vi "XLP80_Globals_Referenzen.vi"() -> ()   [LabVIEW 2021]
uses:
  XLP80_GUI_V001.llb/XLP80_GUI_TDefClusterPandID_Gen2_FM1.ctl
  XLP80_GUI_V001.llb/XLP80_GUI_TDefClusterPandID_Gen2_FM2.ctl
panel:
  in  "References":enum32{"Values", "ModeA", "Mode B", "Display"}(tab)
  in  "AI Values":refnum<vi>
  in  "DI Values":refnum<vi>
  in  "CAN WriteA Values":refnum<vi>
  in  "Listbox TestmodeA ReadCAN":refnum<vi>
  in  "Ref_CAN WriteA Names":refnum<vi>
  in  "Ref_Maxs Alarm":refnum<vi>
  in  "Ref_Names Alarm":refnum<vi>
  in  "Ref Listbox Alarm":refnum<vi>
  in  "Ref_Values Alarm":refnum<vi>
  in  "Ref_Units Alarm":refnum<vi>
  in  "Ref_Mins Alarm":refnum<vi>
  in  "Ref_Maxs Shutdown":refnum<vi>
  in  "Ref_Names Shutdown":refnum<vi>
  in  "Ref Listbox Shutdown":refnum<vi>
  in  "Ref_Values Shutdown":refnum<vi>
  in  "Ref_Units Shutdown":refnum<vi>
  in  "Ref_Mins Shutdown":refnum<vi>
  in  "Ref_Maxs Operational Mode":refnum<vi>
  in  "Ref_Names Operational Mode":refnum<vi>
  in  "Ref Listbox Operational Mode":refnum<vi>
  in  "Ref_Values Operational Mode":refnum<vi>
  in  "Ref_Units Operational Mode":refnum<vi>
  in  "Ref_Mins Operational Mode":refnum<vi>
  in  "Ref_Maxs Precond":refnum<vi>
  in  "Ref_Units Precond":refnum<vi>
  in  "Ref_Mins Precond":refnum<vi>
  in  "Ref_Names Precond":refnum<vi>
  in  "Ref_Values Precond":refnum<vi>
  in  "Ref_Maxs Power Management":refnum<vi>
  in  "Ref_Units Power Management":refnum<vi>
  in  "Ref_Mins Power Management":refnum<vi>
  in  "Ref_Maxs Basis Funktion":refnum<vi>
  in  "Ref_Units Basis Funktion":refnum<vi>
  in  "Ref_Mins Basis Funktion":refnum<vi>
  in  "Ref_Maxs HV&Software":refnum<vi>
  in  "Ref_Names Power Management":refnum<vi>
  in  "Ref Listbox Power Management":refnum<vi>
  in  "Ref_Values Power Management":refnum<vi>
  in  "Ref_Names Basis Funktion":refnum<vi>
  in  "Ref Listbox Basis Funktion":refnum<vi>
  in  "Ref_Values Basis Funktion":refnum<vi>
  in  "Ref_Names HV&Software":refnum<vi>
  in  "Ref Listbox HV&Software":refnum<vi>
  in  "Ref_Values HV&Software":refnum<vi>
  in  "Listbox TestmodeB ReadCAN":refnum<vi>
  in  "Ref_Units HV&Software":refnum<vi>
  in  "Ref_Mins HV&Software":refnum<vi>
  out "ExposureTime":refnum<vi>
  in  "P&ID_GEN2_FM1":refnum<vi>
  in  "Messages":refnum<vi>
  in  "GlobalStateTab":refnum<vi>
  in  "AutoTabCtl":refnum<vi>
  in  "ManTabCtl":refnum<vi>
  in  "P&ID_GEN2_FM2":refnum<vi>
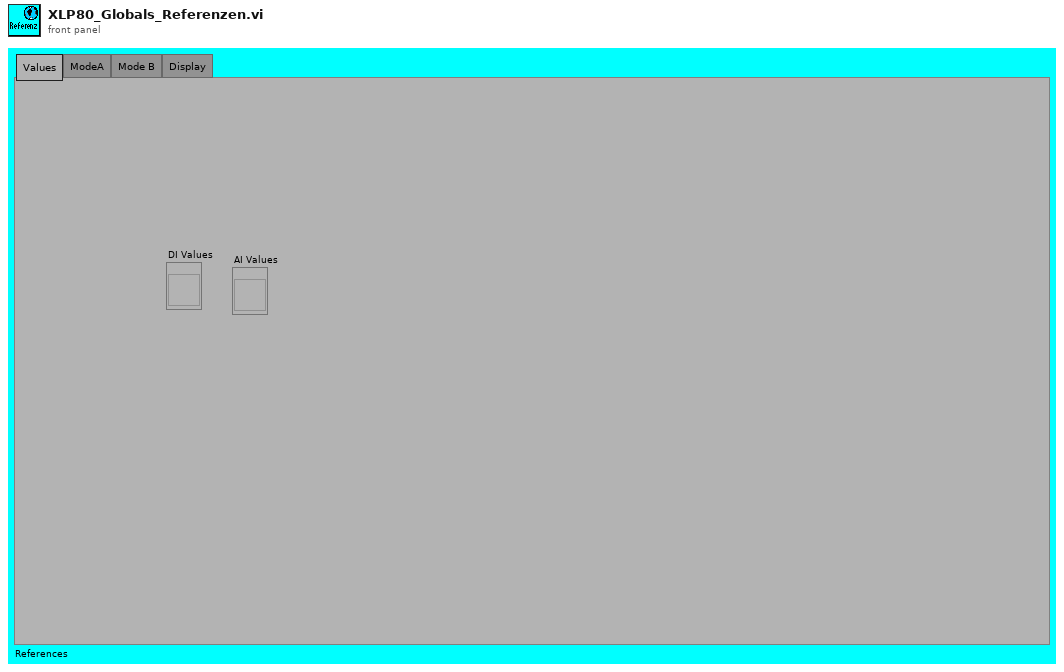
[diagram p1: front panel]
diagram:
